vi "StringToSGL[](cast).vi"(1 "String":string) -> (0 "SGL[]":sgl[](array[numeric]) format="%.2f")   [LabVIEW 2012]
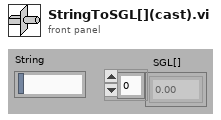
[diagram p1: front panel]
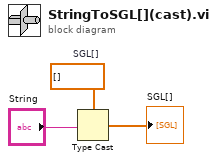
[diagram p0: block diagram]
diagram:
  w2 = sgl[] []  # SGL[]
  n1 = Type Cast(type=w2, x="String") -> (*(type *) &x=→"SGL[]":sgl[])
